vi "Registration_VI.vi"(8 "error in (no error)":errorcluster, 11 "Class 2 in":refnum<class "Panel2.lvclass">) -> (0 "error out":errorcluster, 2 "Core_Reference_VI out":refnum<vi>, 3 "Class 2 out":refnum<class "Panel2.lvclass">)   [LabVIEW 2021, in "Panel2.lvclass"]
uses:
  Panel2.lvclass
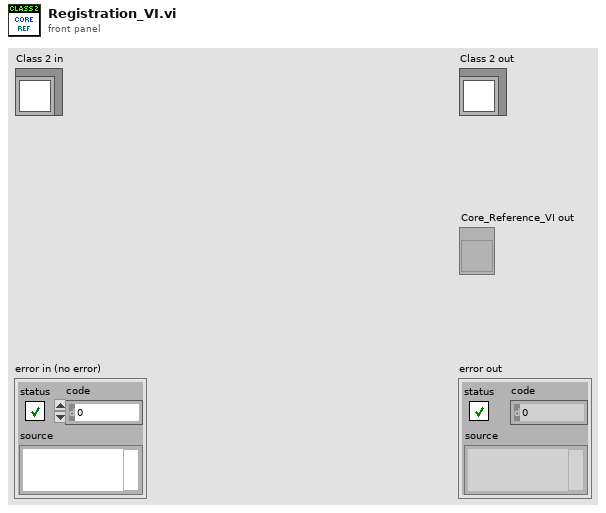
[diagram p1: front panel]
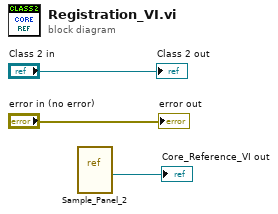
[diagram p0: block diagram]
diagram:
  n1 = vi-ref "Sample_Panel_2.vi"() -> (→"Core_Reference_VI out":refnum<vi>)
  "error out" <- "error in (no error)"
  "Class 2 out" <- "Class 2 in"
